vi "WriteAppConfigRequest.vi"(8 "error in (no error)":errorcluster, 10 "AppConfigXML":string, 11 "ModuleID":i32=-1) -> (0 "error out":errorcluster)   [LabVIEW 2014, in "AppModule.lvlib"]
uses:
  AppModule.lvlib
  clEventType.ctl
  <vilib>/Utility/error.llb/Error Cluster From Error Code.vi
  <vilib>/ErrorRing/Error Ring.xnode
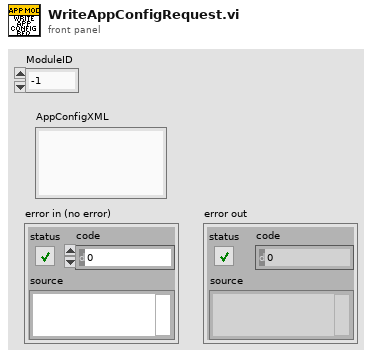
[diagram p1: front panel]
types:
  T1 = typedef "AppModule.lvlib/clRequestEvents.ctl" = cluster{"StopRequest":refnum<user-event>, "PathToINI":refnum<user-event>, " LoadPlugin":refnum<user-event>, "OpenAppConfig":refnum<user-event>, "WriteInputData":refnum<user-event>, "ReadInputData":refnum<user-event>, "GetAppOutput":refnum<user-event>, "WriteEvtConfig":refnum<user-event>, "WriteBcAppInfo":refnum<user-event>, "ReadBcAppInfo":refnum<user-event>, "AggregateRequest":refnum<user-event>, "WriteAppConfig":refnum<user-event>, "ReadAppConfig":refnum<user-event>, "CalcAppOutput":refnum<user-event>, "ShowPanel":refnum<user-event>}
  T2 = typedef "AppModule.lvlib/clEventType.ctl" = cluster{"ModuleID":i32, "Data":variant}
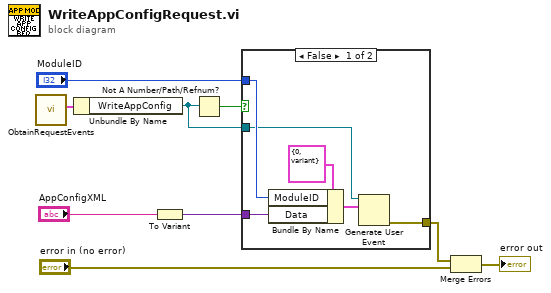
[diagram p0: block diagram]
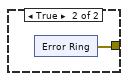
[diagram p2: hidden frame]
diagram:
  n1 = call "ObtainRequestEvents.vi"() -> ("clRequestEvents"=w9:T1)  [unwired: 10 in, 1 out]
  n2 = Unbundle By Name(w9) -> ("WriteAppConfig"=w6:refnum<user-event>)
  n3 = To Variant(anything="AppConfigXML") -> (Variant=w1:variant)
  n4 = Not A Number/Path/Refnum?(number/path/refnum=w6) -> (NaN/Path/Refnum?=w8:bool)
  n5 = case shown="False" w8 {
    tunnel: "ModuleID" -> [w14 _]
    tunnel: w6 -> [w11 _]
    tunnel: w1 -> [w13 _]
    tunnel: [w10 w16] -> w3
    frame False {
      n6 = Bundle By Name(cluster=T2 {"ModuleID"=0, "Data"=variant} ("clEventType"), "ModuleID"=w14, "Data"=w13) -> (w12:T2)
      n7 = Generate User Event(user event=w11, event data cluster=w12) -> (error out=w10:errorcluster)  [unwired: 2 in, 1 out]
    }
    frame True {
      n8 = xnode "Error Ring"() -> ("error out"=w16:errorcluster)
    }
  }
  n9 = Merge Errors(w3, "error in (no error)") -> (→"error out":errorcluster)
